vi "Node - Read Imported Channels Table.vi"(8 "error in (no error)":errorcluster, 11 "Compiled.Settings In":T1) -> (0 "error out":errorcluster, 3 "Compiled.Settings Out":T1)   [LabVIEW 2016, in "PXImc Custom Device System Explorer.lvlib"]
uses:
  PXImc Custom Device System Explorer.lvlib
  Shared/Compiled.Settings.ctl
  <vilib>/NI Veristand/VeriStand Data/Byte Buffer/Byte Buffer.lvclass
  PXImc Router/Controls/Target Type.ctl
  PXImc Router/Controls/Router - Configuration.ctl
  PXImc Router/Controls/Router/Node Block R-W Properties.ctl
  PXImc Router/Controls/Router/Block Properties.ctl
  PXImc Router/Controls/Router/Router - PXImc Properties.ctl
  PXImc Router/Controls/Router/Router - PXImc Card Properties.ctl
  PXImc Router/Controls/Node Data.ctl
  PXImc Router/Controls/Node/Node - PXImc Parameters.ctl
  PXImc Router/Controls/Node/Node - Writer Data.ctl
  PXImc Router/Controls/Node/Node Ch Properties.ctl
  PXImc Router/Controls/Data Type.ctl
  PXImc Router/Controls/Node/Node - Readers Data.ctl
  PXImc Router/Controls/Node/Node - Reader Data.ctl
  <vilib>/Utility/file.llb/Read Delimited Spreadsheet (string).vi
  PXImc Router/PXImc Router.lvlib
  Shared/PXImc Custom Device Shared.lvlib
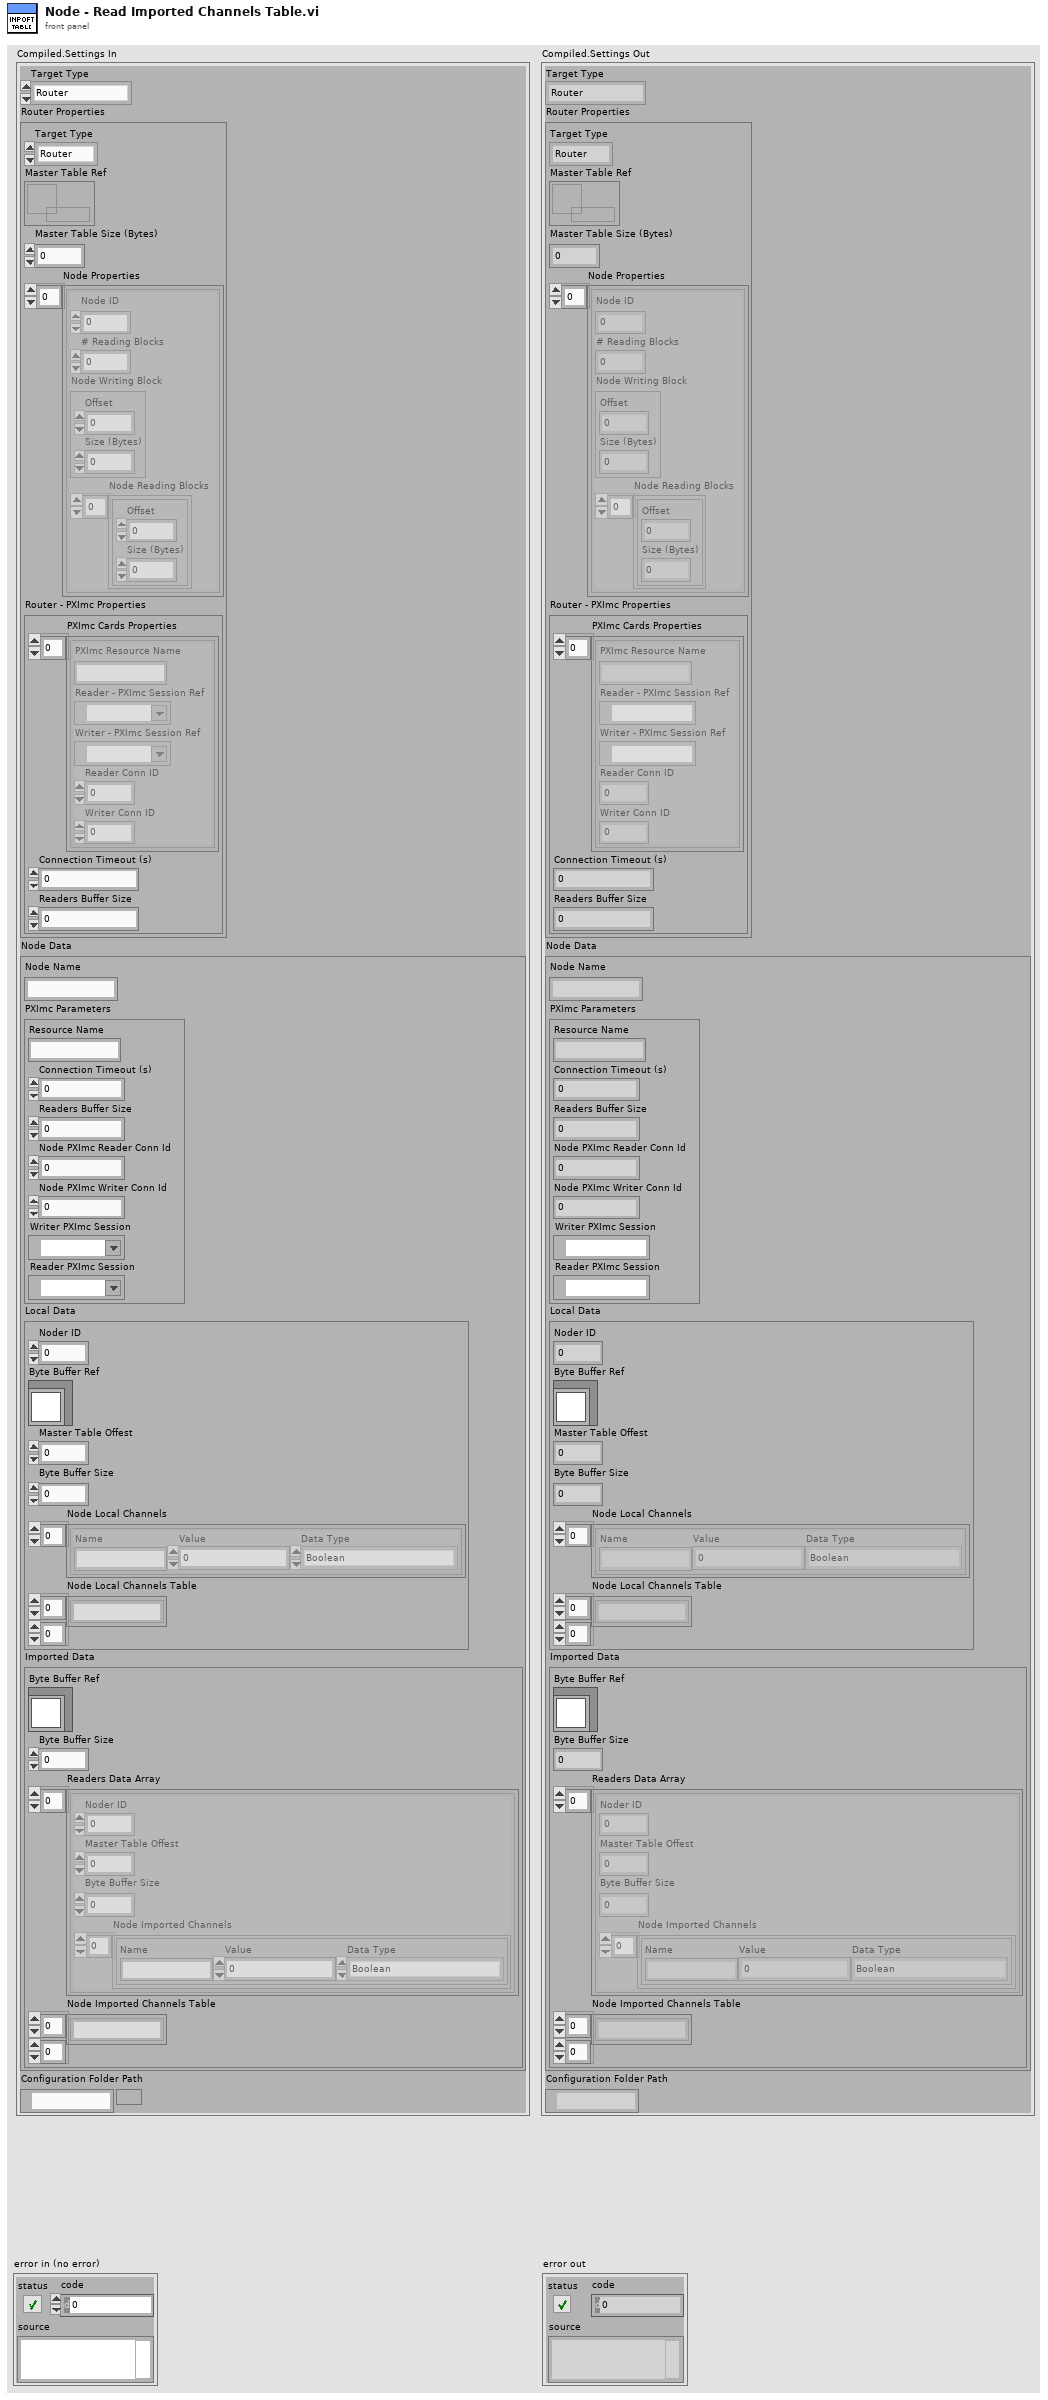
[diagram p1: front panel]
types:
  T1 = typedef "PXImc Custom Device Shared.lvlib/Compiled.Settings.ctl" = cluster{"Target Type":T2, "Router Properties":T3, "Node Data":T8, "Configuration Folder Path":path}
  T2 = typedef "PXImc Router.lvlib/Target Type.ctl" = enum16{"Router", "Node"}
  T3 = typedef "PXImc Router.lvlib/Router - Configuration.ctl" = cluster{"Target Type":T2, "Master Table Ref":refnum<data-value>, "Master Table Size (Bytes)":u32, "Node Properties":T4[], "Router - PXImc Properties":T6}
  T4 = typedef "PXImc Router.lvlib/Node Block R-W Properties.ctl" = cluster{"Node ID":u32, "# Reading Blocks":u32, "Node Writing Block":T5, "Node Reading Blocks":T5[]}
  T5 = typedef "PXImc Router.lvlib/Block Properties.ctl" = cluster{"Offset":u32, "Size (Bytes)":u32}
  T6 = typedef "PXImc Router.lvlib/Router - PXImc Properties.ctl" = cluster{"PXImc Cards Properties":T7[], "Connection Timeout (s)":dbl, "Readers Buffer Size":u64}
  T7 = typedef "PXImc Router.lvlib/Router - PXImc Card Properties.ctl" = cluster{"PXImc Resource Name":string, "Reader - PXImc Session Ref":refnum<k21>, "Writer - PXImc Session Ref":refnum<k21>, "Reader Conn ID":u16, "Writer Conn ID":u16}
  T8 = typedef "PXImc Router.lvlib/Node Data.ctl" = cluster{"Node Name":string, "PXImc Parameters":T9, "Local Data":T10, "Imported Data":T13}
  T9 = typedef "PXImc Router.lvlib/Node - PXImc Parameters.ctl" = cluster{"Resource Name":string, "Connection Timeout (s)":dbl, "Readers Buffer Size":u64, "Node PXImc Reader Conn Id":u16, "Node PXImc Writer Conn Id":u16, "Writer PXImc Session":refnum<k21>, "Reader PXImc Session":refnum<k21>}
  T10 = typedef "PXImc Router.lvlib/Node - Writer Data.ctl" = cluster{"Noder ID":u32, "Byte Buffer Ref":refnum<class "Byte Buffer.lvclass">, "Master Table Offest":u32, "Byte Buffer Size":u32, "Node Local Channels":T11[], "Node Local Channels Table":string[][]}
  T11 = typedef "PXImc Router.lvlib/Node Ch Properties.ctl" = cluster{"Name":string, "Value":dbl, "Data Type":T12}
  T12 = typedef "PXImc Router.lvlib/Data Type.ctl" = enum16{"Boolean", "SGL", "DBL", "I8", "I16", "I32", "I64", "U8", "U16", "U32", "U64"}
  T13 = typedef "PXImc Router.lvlib/Node - Readers Data.ctl" = cluster{"Byte Buffer Ref":refnum<class "Byte Buffer.lvclass">, "Byte Buffer Size":u64, "Readers Data Array":T14[], "Node Imported Channels Table":string[][]}
  T14 = typedef "PXImc Router.lvlib/Node - Reader Data.ctl" = cluster{"Noder ID":u32, "Master Table Offest":u32, "Byte Buffer Size":u64, "Node Imported Channels":T11[]}
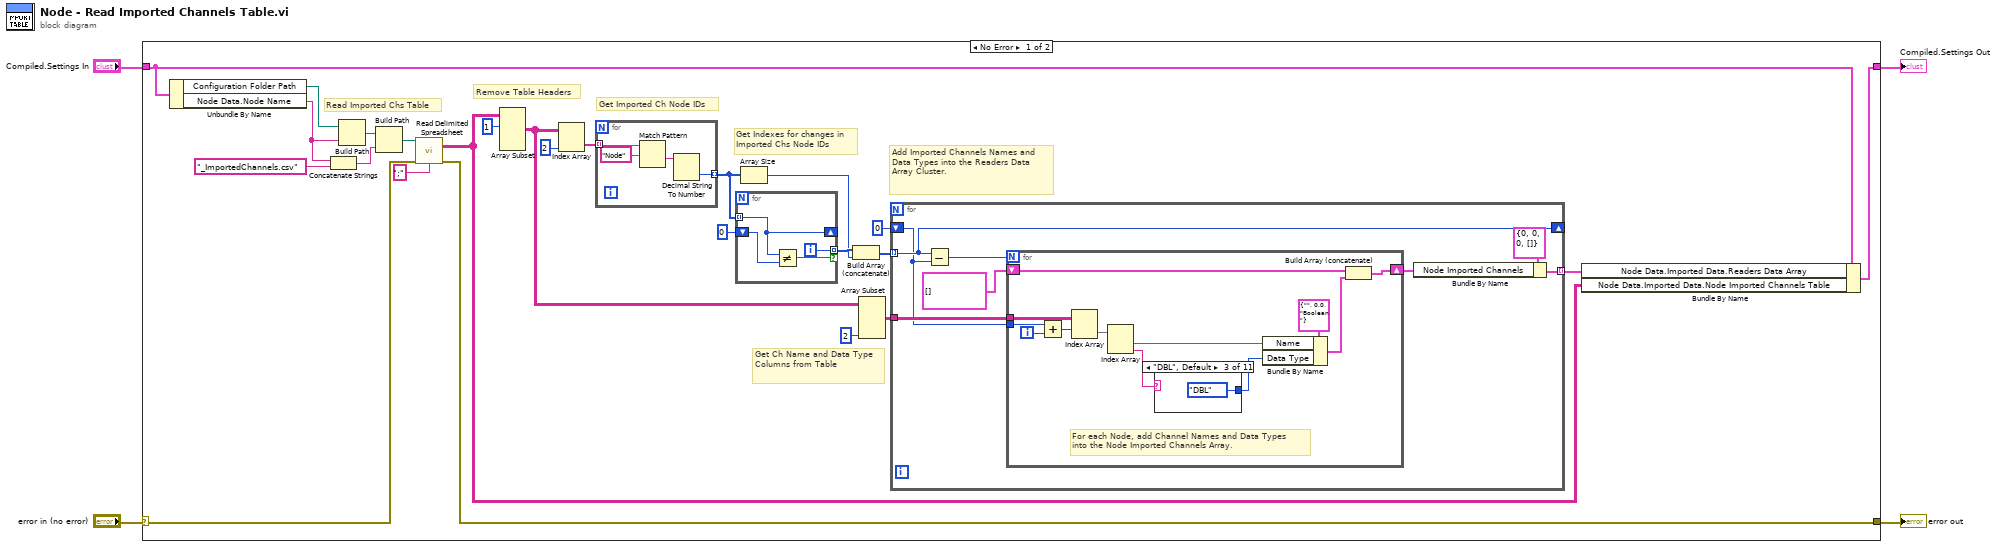
[diagram p0: block diagram]
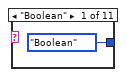
[diagram p2: hidden frame]
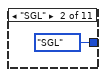
[diagram p3: hidden frame]
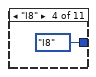
[diagram p4: hidden frame]
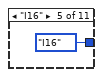
[diagram p5: hidden frame]
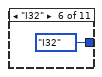
[diagram p6: hidden frame]
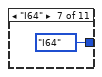
[diagram p7: hidden frame]
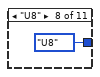
[diagram p8: hidden frame]
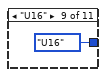
[diagram p9: hidden frame]
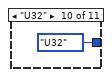
[diagram p10: hidden frame]
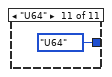
[diagram p11: hidden frame]
diagram:
  n1 = case shown="No Error" "error in (no error)" {
    selector: "error in (no error)" -> [w20 w69]
    tunnel: "Compiled.Settings In" -> [w25 w70]
    tunnel: [w26 w70] -> w3
    tunnel: [w19 w69] -> w1
    frame No Error {
      # "Add Imported Channels Names and Data Types into the Readers Data Array Cluster."
      # "Get Ch Name and Data Type Columns from Table"
      # "Read Imported Chs Table"
      # "Get Indexes for changes in \nImported Chs Node IDs"
      # "Get Imported Ch Node IDs"
      # "Remove Table Headers"
      n2 = Unbundle By Name(w25) -> ("Configuration Folder Path"=w24:path, "Node Data.Node Name"=w6:string)
      n3 = Concatenate Strings(w6, "_ImportedChannels.csv" ("name or relative path")) -> (w22:string)
      n4 = Build Path(base path=w24, name or relative path=w6) -> (appended path=w29:path)
      n5 = Build Path(base path=w29, name or relative path=w22) -> (appended path=w28:path)
      n6 = call-poly <vilib>:"Read Delimited Spreadsheet.vi"("file path (dialog if empty)"=w28, "error in (no error)"=w20, "delimiter (\\t)"=";" ("delimiter (\\t)")) -> ("all rows"=w5:string[][], "error out"=w19:errorcluster)  [unwired: 7 in, 4 out]
      n7 = Array Subset(array=w5, index (row)=1 ("index")) -> (w16:string[][])  [unwired: 3 in]
      n8 = Index Array(array=w16, index (col)=2 ("disabled index (col)")) -> (element=w17:string[])  [unwired: 1 in]
      n9 = for {
        tunnel: w17 -> [w68] mode=indexing
        tunnel: [w65] -> w9 mode=indexing
        n10 = Match Pattern(string=w68, regular expression="Node") -> (after substring=w66:string)  [unwired: 1 in, 3 out]
        n11 = Decimal String To Number(string=w66) -> (number=w65:i32)  [unwired: 2 in, 1 out]
      }
      n12 = for {
        tunnel: w9 -> [w63] mode=indexing
        shift-right: [w63] -> _
        shift-left: 0 -> [w64]
        tunnel: [w61] -> w10 mode=indexing if=w62
        i -> [w61]
        n13 = Not Equal?(x=w63, y=w64) -> (x != y?=w62:bool)
      }
      n14 = Array Size(array=w9) -> (size(s)=w7:i32)
      n15 = Build Array (concatenate)(w10, w7) -> (w8:i32[])
      n16 = Array Subset(array=w16, length (col)=2 ("length")) -> (w14:string[][])  [unwired: 3 in]
      n17 = for {
        tunnel: w8 -> [w32] mode=indexing
        tunnel: [w33] -> w13 mode=indexing
        shift-right: [w32] -> _
        shift-left: 0 -> [w31]
        tunnel: w14 -> [w37]
        n18 = Subtract(x=w32, y=w31) -> (x-y=w30:i32)
        n19 = for {
          N: w30 -> [_]
          tunnel: w31 -> [w39]
          shift-right: [w40] -> w34
          shift-left: T11[] [] ("Node Local Channels") -> [w41]
          tunnel: w37 -> [w44]
          i -> [w38]
          # "For each Node, add Channel Names and Data Types \ninto the Node Imported Channels Array."
          n20 = Add(x=w39, y=w38) -> (x+y=w45:i32)
          n21 = Index Array(array=w44, index (row)=w45) -> (element=w48:string[])  [unwired: 1 in]
          n22 = Index Array(array=w48) -> (element #1=w47:string, element #2=w46:string)  [unwired: 2 in]
          n23 = case shown="\"DBL\", Default" w46 {
            tunnel: [Data_Type."Boolean" ("Data Type") Data_Type."SGL" ("Data Type") Data_Type."DBL" ("Data Type") Data_Type."I8" ("Data Type") Data_Type."I16" ("Data Type") Data_Type."I32" ("Data Type") Data_Type."I64" ("Data Type") Data_Type."U8" ("Data Type") Data_Type."U16" ("Data Type") Data_Type."U32" ("Data Type") Data_Type."U64" ("Data Type")] -> w49
            frame "Boolean" {
            }
            frame "SGL" {
            }
            frame "DBL", Default {
            }
            frame "I8" {
            }
            frame "I16" {
            }
            frame "I32" {
            }
            frame "I64" {
            }
            frame "U8" {
            }
            frame "U16" {
            }
            frame "U32" {
            }
            frame "U64" {
            }
          }
          n24 = Bundle By Name(cluster=T11 {"Name"="", "Value"=0.0, "Data Type"=enum."Boolean"} ("Node Ch Properties"), "Name"=w47, "Data Type"=w49) -> (w42:T11)
          n25 = Build Array (concatenate)(w41, w42) -> (w40:T11[])
        }
        n26 = Bundle By Name(cluster=T14 {"Noder ID"=0, "Master Table Offest"=0, "Byte Buffer Size"=0, "Node Imported Channels"=[]} ("Reader Data"), "Node Imported Channels"=w34) -> (w33:T14)
      }
      n27 = Bundle By Name(cluster=w25, "Node Data.Imported Data.Readers Data Array"=w13, "Node Data.Imported Data.Node Imported Channels Table"=w5) -> (w26:T1)
    }
    frame Error {
    }
  }
  "Compiled.Settings Out" <- w3
  "error out" <- w1
